vi "check if do another checkpoint.vi"(8 "error in (no error)":errorcluster, 11 "Autofocus in":refnum<class "Autofocus.lvclass">) -> (0 "error out":errorcluster, 2 "do more checkpoints?":bool, 3 "Autofocus out":refnum<class "Autofocus.lvclass">)   [LabVIEW 2012, in "Autofocus.lvclass"]
uses:
  Autofocus.lvclass
  Autofocus.lvclass/Autofocus.ctl
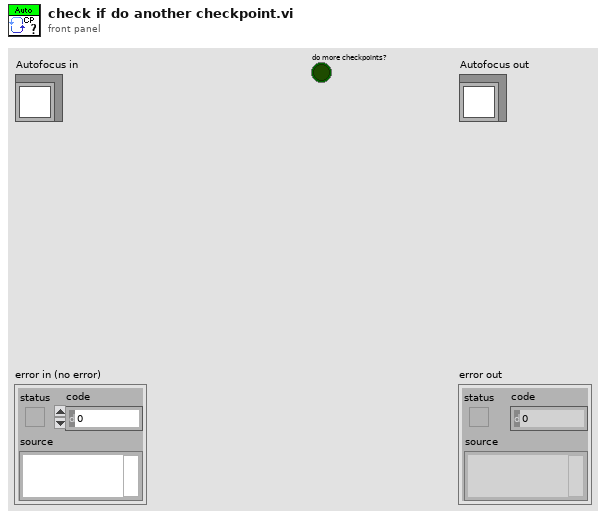
[diagram p1: front panel]
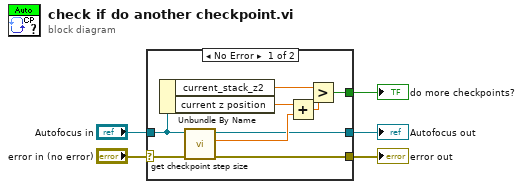
[diagram p0: block diagram]
diagram:
  n1 = case shown="No Error" "error in (no error)" {
    selector: "error in (no error)" -> [w14 w16]
    tunnel: [w13 w16] -> w4
    tunnel: [w9 w15] -> w2
    tunnel: "Autofocus in" -> [w10 w15]
    tunnel: [w6 _] -> w1
    frame No Error {
      n2 = Unbundle By Name(w10) -> ("current_stack_z2"=w7:dbl[unit], "current z position"=w8:dbl[unit])
      n3 = call-dynamic "get checkpoint step size.vi"("error in (no error)"=w14, "Autofocus in"=w10) -> ("error out"=w13:errorcluster, "checkpoint stepsize"=w11:dbl[unit], "Autofocus out"=w9:refnum<class "Autofocus.lvclass">)  [unwired: 7 in]
      n4 = Add(x=w8, y=w11) -> (x+y=w12:dbl[unit])
      n5 = Greater?(x=w7, y=w12) -> (0:w6:bool)
    }
    frame Error {
    }
  }
  "error out" <- w4
  "Autofocus out" <- w2
  "do more checkpoints?" <- w1
